vi "Main.vi"() -> ()   [LabVIEW 2014, in "ConfigurableQMH.lvlib"]
doc: "This template is based off of the Queued Message Handler design pattern and the Queued Message Handler project template that ships with LabVIEW.\n\nThe main difference is that the queue is private to this module and communication between modules is performed via Broadcast and Request events.\n\nRequest events are wrapped in public API methods and are handled in the Event Handling Loop (EHL) of this VI. Any module can register for Broadcast events sent by this module. The EHL generates messages based on user interface actions.\n\nThe Message Handling Loop (MHL) processes messages generated by the EHL, or by other messages. The messages are string values, so new messages can be added easily to the Message Cases case structure in the MHL. Each message cluster can also provide an optional value for Message Data, which is a variant that can be converted to whatever message-specific data is required.\n_____\nBased on Delacor QMH Project Template 4.0.0.47."
uses:
  ConfigurableQMH.lvlib
  <vilib>/Delacor/Delacor QMH/Libraries/Cloneable Module Admin_class/Delacor_lib_QMH_Cloneable Module Admin.lvclass
  <vilib>/LabVIEW Open Source/Configuration Manager/Manager/ConfigManager.lvclass
  <vilib>/LabVIEW Open Source Project/Unicity/UniqueName/UniqueNameClass/UniqueName.lvclass
  ModuleConfiguration--Cluster.ctl
  Module Data--cluster.ctl
  <vilib>/Delacor/Delacor QMH/Libraries/Cloneable Module Admin_class/Delacor_lib_QMH_Cloneable Module Admin.lvclass/Delacor_lib_QMH_Cloneable Module Admin.ctl
  Stop Argument--cluster.ctl
  <vilib>/Delacor/Delacor QMH/Libraries/Module Admin_class/Delacor_lib_QMH_Module Admin.lvclass/Delacor_lib_QMH_Module Admin.ctl
  GetQualifiedName Argument--cluster.ctl
  GetQualifiedName (Reply Payload)--cluster.ctl
  GetConfiguration Argument--cluster.ctl
  GetConfiguration (Reply Payload)--cluster.ctl
  Modify Configuration Argument--cluster.ctl
  <vilib>/Utility/miscctls.llb/LVPointTypeDef.ctl
  <vilib>/LabVIEW Open Source Project/Unicity/UniqueName/UniqueNameClass/UniqueName.lvclass/UniqueName.ctl
  <vilib>/Delacor/Delacor QMH/Libraries/Cloneable Module Admin_class/Delacor_lib_QMH_Get Module ID.vi
  <vilib>/Delacor/Delacor QMH/Libraries/Module Admin_class/Delacor_lib_QMH_Get External Launch.vi
  <vilib>/Delacor/Delacor QMH/Libraries/Message Queue_class/Delacor_lib_QMH_Enqueue Message (Single).vi
  <vilib>/Utility/error.llb/Error Cluster From Error Code.vi
  <vilib>/ErrorRing/Error Ring.xnode
  <vilib>/Delacor/Delacor QMH/Libraries/Message Queue_class/Delacor_lib_QMH_Message Queue.lvclass
  Clone Registration/Clone Registration.lvlib
panel:
  in  "SubModule Name":string
  in  "Launch SubModule":bool
  out "Initial Configuration":T1
  out "Current Configuration":T1
  in  "Self":refnum<class "UniqueName.lvclass">
  in  "CfgManager":refnum<class "ConfigManager.lvclass">
  in  "Simulate MHL Error":bool
  in  "Simulate EHL Error":bool
  out "error out":errorcluster
  in  "Module Admin":refnum<class "Delacor_lib_QMH_Cloneable Module Admin.lvclass">
  out "Status":string
  # "Do not modify these nodes"
  # "This template is for the a Configurable  Delacor Queued Message Handler design pattern.\n\nSee the block diagram for more information on how to use this template.\nOther QMH Modules communicate with this Module via its Public API (wrappers for its Request Events).\n\nThis Module communicates with other Modules via its Broadcast Events.\nAny module that wants to get these messages, just registers for this module's Broadcast events."
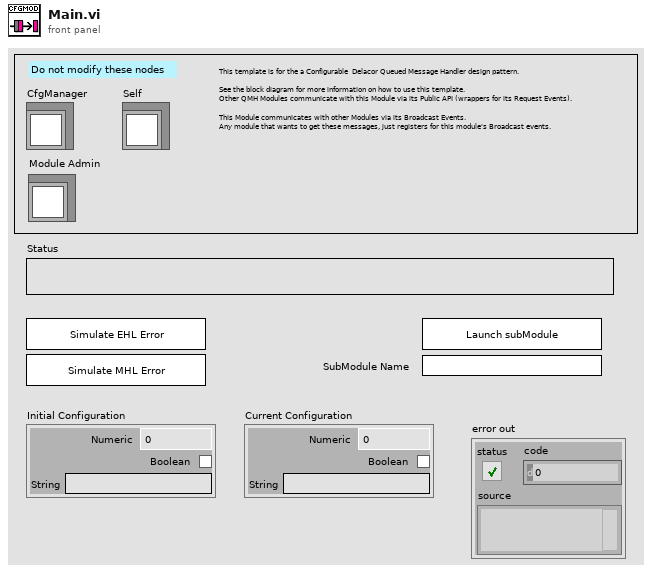
[diagram p1: front panel]
types:
  T1 = typedef "ConfigurableQMH.lvlib/ModuleConfiguration--Cluster.ctl" = cluster{"Numeric":dbl, "Boolean":bool, "String":string}
  T2 = typedef "ConfigurableQMH.lvlib/Module Data--cluster.ctl" = cluster{"Status":string, "CfgManager":refnum<class "ConfigManager.lvclass">, "Self":refnum<class "UniqueName.lvclass">, "Submodules":i32[]}
  T3 = typedef "ConfigurableQMH.lvlib/Request Events--cluster.ctl" = cluster{"Stop Module":refnum<user-event>, "Show Panel":refnum<user-event>, "Hide Panel":refnum<user-event>, "Show Diagram":refnum<user-event>, "Get Module Execution Status":refnum<user-event>, "GetQualifiedName":refnum<user-event>, "GetConfiguration":refnum<user-event>, "Modify Configuration":refnum<user-event>}
  T4 = enum32{"invalid lock state", "Not Locked", "Locked (No Password)", "Password-protected"}
  T5 = typedef "ConfigurableQMH.lvlib/Stop Argument--cluster.ctl" = cluster{"Origin":string, "Module ID":i32, "Exit via Stop Module Req?":bool, "Wait for Module to stop?":bool}
  T6 = typedef "ConfigurableQMH.lvlib/GetQualifiedName Argument--cluster.ctl" = cluster{"Module ID":i32, "Fully Qualified Name":string, "Wait Notifier":refnum<notifier>}
  T7 = typedef "ConfigurableQMH.lvlib/GetConfiguration Argument--cluster.ctl" = cluster{"Module ID":i32, "Wait Notifier":refnum<notifier>}
  T8 = typedef "ConfigurableQMH.lvlib/Modify Configuration Argument--cluster.ctl" = cluster{"Module ID":i32, "Configuration":T1}
  T9 = typedef "LVPointTypeDef.ctl" = cluster{"Horizontal":i16, "Vertical":i16}
  T10 = enum32{"Invalid", "Standard", "Closed", "Hidden", "Minimized", "Maximized"}
  T11 = typedef "ConfigurableQMH.lvlib/GetQualifiedName (Reply Payload)--cluster.ctl" = cluster{"Fully Qualified Name":string, "GetQualifiedName_error":errorcluster}
  T12 = typedef "ConfigurableQMH.lvlib/GetConfiguration (Reply Payload)--cluster.ctl" = cluster{"Configuration":T1, "GetConfiguration_error":errorcluster}
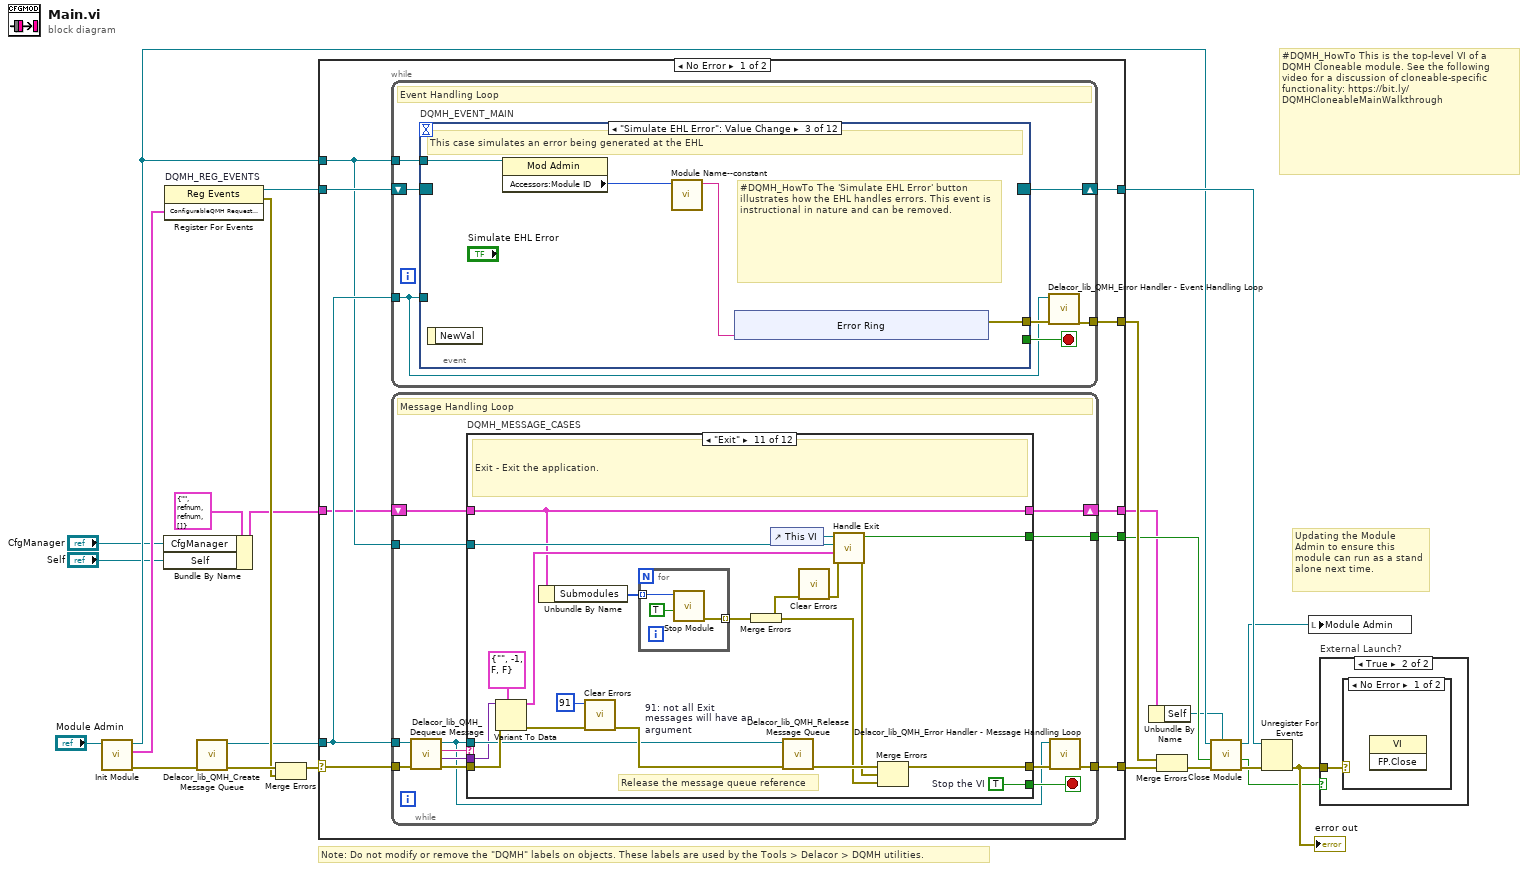
[diagram p0: block diagram]
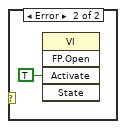
[diagram p3: hidden frame]
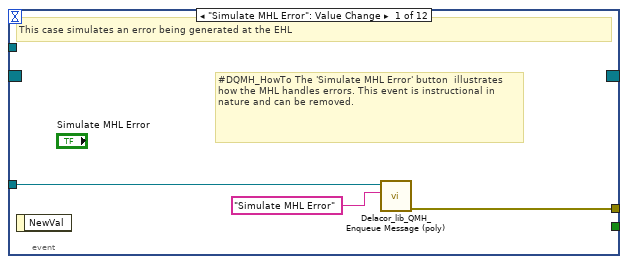
[diagram p4: hidden frame]
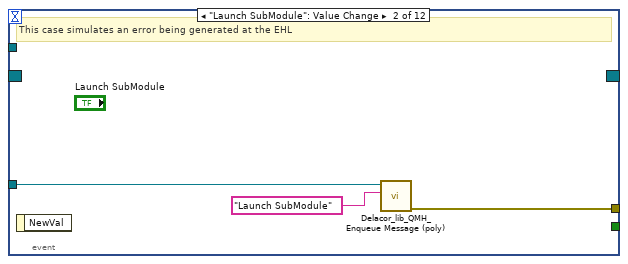
[diagram p5: hidden frame]
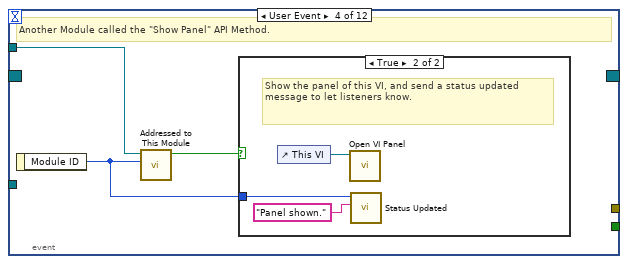
[diagram p6: hidden frame]
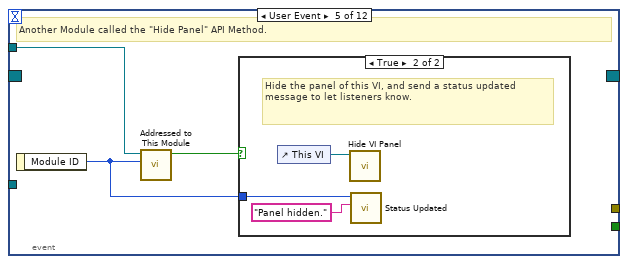
[diagram p8: hidden frame]
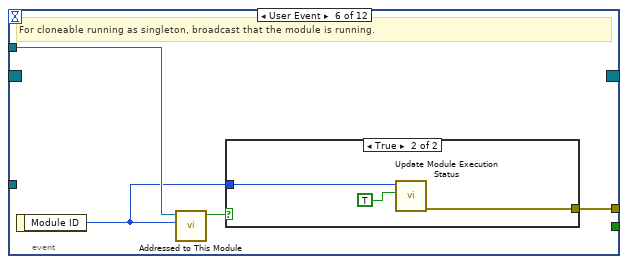
[diagram p10: hidden frame]
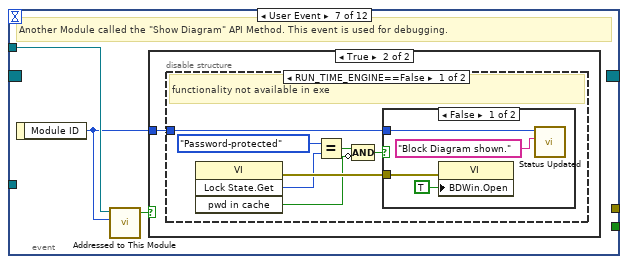
[diagram p12: hidden frame]
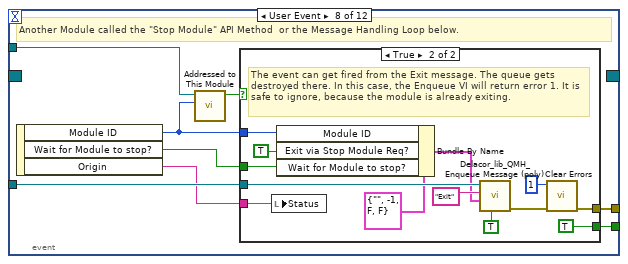
[diagram p16: hidden frame]
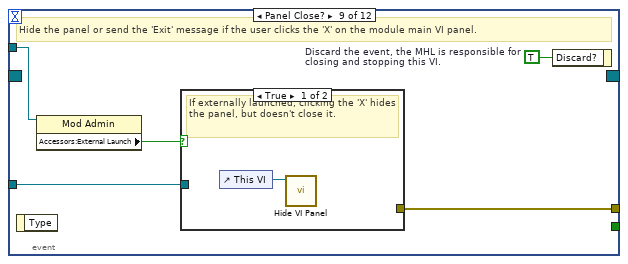
[diagram p18: hidden frame]
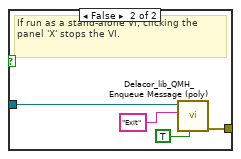
[diagram p19: hidden frame]
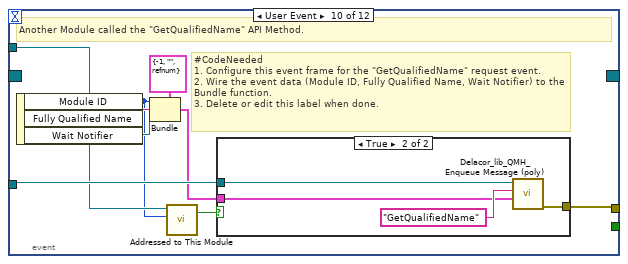
[diagram p20: hidden frame]
diagram:
  # "#DQMH_HowTo This is the top-level VI of a DQMH Cloneable module. See the following video for a discussion of cloneable-specific functionality: https://bit.ly/DQMHCloneableMainWalkthrough"
  # "Note: Do not modify or remove the \"DQMH\" labels on objects. These labels are used by the Tools > Delacor > DQMH utilities."
  # "Updating the Module Admin to ensure this module can run as a stand alone next time."
  n1 = call "Init Module.vi"("Cloneable Module Admin in"="Module Admin") -> ("error out"=w21:errorcluster, "ConfigurableQMH Request Events"=w13:T3, "Cloneable Module Admin out"=w10:refnum<class "Delacor_lib_QMH_Cloneable Module Admin.lvclass">)  [unwired: 8 in]
  n2 = Bundle By Name(cluster=T2 {"Status"="", "CfgManager"=refnum, "Self"=refnum, "Submodules"=[]} ("Data Cluster"), "CfgManager"="CfgManager", "Self"="Self") -> (w4:T2)
  n3 = register-events "DQMH_REG_EVENTS"(w13) -> (reference out=w14:refnum<event-registration>, error out=w16:errorcluster)  [unwired: 2 in]
  n4 = call <vilib>:"Delacor_lib_QMH_Create Message Queue.vi"("error in (no error)"=w21) -> ("error out"=w18:errorcluster, "Message Queue out"=w12:refnum<class "Delacor_lib_QMH_Message Queue.lvclass">)  [unwired: 9 in]
  n5 = Merge Errors(w18, w16) -> (w17:errorcluster)
  n6 = case shown="No Error" w17 {
    selector: w17 -> [w32 w339]
    tunnel: [w34 w339] -> w22
    tunnel: [w31 w338] -> w15
    tunnel: w14 -> [w30 w338]
    tunnel: w12 -> [w29 _]
    tunnel: [w33 _] -> w23
    tunnel: w10 -> [w28 w334]
    tunnel: [w27 _] -> w8
    tunnel: w4 -> [w26 w331]
    tunnel: [w25 w331] -> w1
    frame No Error {
      n7 = while {
        tunnel: w29 -> [w35]
        shift-right: [w38] -> w31
        shift-left: w30 -> [w39]
        tunnel: [w40] -> w33
        tunnel: w28 -> [w36]
        stop <- w37 stop-if-true
        # "Event Handling Loop"
        n8 = event "DQMH_EVENT_MAIN" shown="[2] \"Simulate EHL Error\": Value Change" {
          selector: w39 -> [_ _ _ _ _ _ _ _ _ _ _ _]
          dyn-events: [_ _ _ _ _ _ _ _ _ _ _ _] -> w38
          timeout: _ -> [_ _ _ _ _ _ _ _ _ _ _ _]
          tunnel: [_ _ _ _ _ _ _ w96 _ _ _ _] -> w37
          tunnel: w35 -> [w43 w46 _ _ _ _ _ w99 w115 w132 w144 w156]
          tunnel: [w44 w47 w51 _ _ w74 _ w100 w118 w127 w139 w151] -> w41
          tunnel: w36 -> [_ _ w50 w60 w66 w72 w79 w98 w116 w130 w142 w154]
          event "Simulate MHL Error": Value Change {
            # "#DQMH_HowTo The 'Simulate MHL Error' button  illustrates how the MHL handles errors. This event is instructional in nature and can be removed."
            # "This case simulates an error being generated at the EHL"
            n9 = event-data() -> ()  [unwired: 1 in, 1 out]
            n10 = call-poly <vilib>:"Delacor_lib_QMH_Enqueue Message (poly).vi"("Message"="Simulate MHL Error", "Message Queue in"=w43) -> ("error out"=w44:errorcluster)  [unwired: 8 in, 1 out]
          }
          event "Launch SubModule": Value Change {
            # "This case simulates an error being generated at the EHL"
            n11 = event-data() -> ()  [unwired: 1 in, 1 out]
            n12 = call-poly <vilib>:"Delacor_lib_QMH_Enqueue Message (poly).vi"("Message"="Launch SubModule", "Message Queue in"=w46) -> ("error out"=w47:errorcluster)  [unwired: 8 in, 1 out]
          }
          event "Simulate EHL Error": Value Change {
            # "#DQMH_HowTo The 'Simulate EHL Error' button  illustrates how the EHL handles errors. This event is instructional in nature and can be removed."
            # "This case simulates an error being generated at the EHL"
            n13 = event-data() -> ()  [unwired: 1 in, 1 out]
            n14 = property class="Mod Admin"(reference=w50) -> ("Accessors:Module ID"=w49:i32)  [unwired: 1 in, 2 out]
            n15 = call "Module Name--constant.vi"("Module ID"=w49) -> ("Module Name"=w48:string)  [unwired: 10 in]
            n16 = xnode "Error Ring"("parameter 0"=w48) -> ("error out"=w51:errorcluster)
          }
          event User Event {
            # "Another Module called the \"Show Panel\" API Method."
            n17 = event-data() -> ("Module ID"=w59:i32)  [unwired: 1 in]
            n18 = call "Addressed to This Module.vi"("Module ID from Argument"=w59, "Module Admin"=w60) -> ("Addressed to this instance?"=w61:bool)  [unwired: 8 in, 1 out]
            n19 = case shown="True" w61 {
              tunnel: w59 -> [_ w62]
              frame False {
              }
              frame True {
                # "Show the panel of this VI, and send a status updated message to let listeners know."
                n20 = control-ref of="This VI"() -> (w64:refnum<vi>)
                n21 = call "Open VI Panel.vi"("VI"=w64) -> ()  [unwired: 10 in, 1 out]
                n22 = call "Status Updated.vi"("Status"="Panel shown." ("format string"), "Module ID"=w62) -> ()  [unwired: 9 in, 1 out]
              }
            }
          }
          event User Event {
            # "Another Module called the \"Hide Panel\" API Method."
            n23 = event-data() -> ("Module ID"=w65:i32)  [unwired: 1 in]
            n24 = call "Addressed to This Module.vi"("Module ID from Argument"=w65, "Module Admin"=w66) -> ("Addressed to this instance?"=w67:bool)  [unwired: 8 in, 1 out]
            n25 = case shown="True" w67 {
              tunnel: w65 -> [_ w68]
              frame False {
              }
              frame True {
                # "Hide the panel of this VI, and send a status updated message to let listeners know."
                n26 = control-ref of="This VI"() -> (w70:refnum<vi>)
                n27 = call "Hide VI Panel.vi"("VI"=w70) -> ()  [unwired: 10 in, 1 out]
                n28 = call "Status Updated.vi"("Status"="Panel hidden." ("format string"), "Module ID"=w68) -> ()  [unwired: 9 in, 1 out]
              }
            }
          }
          event User Event {
            # "For cloneable running as singleton, broadcast that the module is running."
            n29 = event-data() -> ("Module ID"=w71:i32)  [unwired: 1 in]
            n30 = call "Addressed to This Module.vi"("Module ID from Argument"=w71, "Module Admin"=w72) -> ("Addressed to this instance?"=w73:bool)  [unwired: 8 in, 1 out]
            n31 = case shown="True" w73 {
              tunnel: [_ w77] -> w74
              tunnel: w71 -> [_ w76]
              frame False {
              }
              frame True {
                n32 = call "Update Module Execution Status.vi"("Running?"=TRUE, "Module ID"=w76) -> ("error out"=w77:errorcluster)  [unwired: 9 in]
              }
            }
          }
          event User Event {
            # "Another Module called the \"Show Diagram\" API Method. This event is used for debugging."
            n33 = event-data() -> ("Module ID"=w78:i32)  [unwired: 1 in]
            n34 = call "Addressed to This Module.vi"("Module ID from Argument"=w78, "Module Admin"=w79) -> ("Addressed to this instance?"=w80:bool)  [unwired: 8 in, 1 out]
            n35 = case shown="True" w80 {
              tunnel: w78 -> [_ w81]
              frame False {
              }
              frame True {
                n36 = disable-structure shown="RUN_TIME_ENGINE==False" {
                  disable-tunnel: w81 -> [w82 _]
                  frame condition #0 (active) {
                    # "functionality not available in exe"
                    n37 = invoke class="VI" method="Lock State.Get"() -> (error out=w88:errorcluster, "Get Lock State"=w87:T4, "pwd in cache"=w84:bool)  [unwired: 4 in, 1 out]
                    n38 = Equal?(x=T4."Password-protected", y=w87) -> (x = y?=w85:bool)
                    n39 = Compound Arithmetic op=AND(w85, invert w84) -> (w83:bool)
                    n40 = case shown="False" w83 {
                      tunnel: w88 -> [w92 _]
                      tunnel: w82 -> [w89 _]
                      frame False {
                        n41 = property class="VI"(error in=w92, "BDWin.Open"=TRUE ("Block Diagram Window:Open")) -> ()  [unwired: 1 in, 2 out]
                        n42 = call "Status Updated.vi"("Status"="Block Diagram shown." ("format string"), "Module ID"=w89) -> ()  [unwired: 9 in, 1 out]
                      }
                      frame True {
                        # "Password-protected VI, and the password is not in the cache. Do not show the diagram."
                      }
                    }
                  }
                  frame condition #1 {
                  }
                }
              }
            }
          }
          event User Event {
            # "Another Module called the \"Stop Module\" API Method  or the Message Handling Loop below."
            n43 = event-data() -> ("Module ID"=w94:i32, "Wait for Module to stop?"=w95:bool, "Origin"=w93:string)  [unwired: 1 in]
            n44 = call "Addressed to This Module.vi"("Module ID from Argument"=w94, "Module Admin"=w98) -> ("Addressed to this instance?"=w97:bool)  [unwired: 8 in, 1 out]
            n45 = case shown="True" w97 {
              tunnel: [_ w112] -> w100
              tunnel: w99 -> [_ w108]
              tunnel: [_ TRUE] -> w96
              tunnel: w95 -> [_ w103]
              tunnel: w94 -> [_ w105]
              tunnel: w93 -> [_ w101]
              frame False {
              }
              frame True {
                # "The event can get fired from the Exit message. The queue gets destroyed there. In this case, the Enqueue VI will return error 1. It is safe to ignore, because the module is already exiting."
                n46 = local write "Status"(w101) -> ()
                n47 = Bundle By Name(cluster=T5 {"Origin"="", "Module ID"=-1, "Exit via Stop Module Req?"=FALSE, "Wait for Module to stop?"=FALSE} ("Stop Argument"), "Module ID"=w105, "Exit via Stop Module Req?"=TRUE, "Wait for Module to stop?"=w103) -> (w102:T5)
                n48 = call-poly <vilib>:"Delacor_lib_QMH_Enqueue Message (poly).vi"("Priority Message? (F)"=TRUE, "Message Data"=w102, "Message"="Exit", "Message Queue in"=w108) -> ("error out"=w113:errorcluster)  [unwired: 6 in, 1 out]
                n49 = call <vilib>:"Clear Errors.vi"("error in (no error)"=w113, "specific error code to clear (0: all)"=1) -> ("error out"=w112:errorcluster)  [unwired: 4 in, 1 out]
              }
            }
          }
          event Panel Close? {
            w117 = TRUE  # Discard the event, the MHL is responsible for closing and stopping this VI.
            # "Hide the panel or send the 'Exit' message if the user clicks the 'X' on the module main VI panel."
            n50 = event-data() -> ()  [unwired: 1 in, 1 out]
            n51 = property class="Mod Admin"(reference=w116) -> ("Accessors:External Launch"=w114:bool)  [unwired: 1 in, 2 out]
            n52 = case shown="True" w114 {
              tunnel: w115 -> [_ w122]
              tunnel: [_ w123] -> w118
              frame True {
                # "If externally launched, clicking the 'X' hides the panel, but doesn't close it."
                n53 = control-ref of="This VI"() -> (w119:refnum<vi>)
                n54 = call "Hide VI Panel.vi"("VI"=w119) -> ()  [unwired: 10 in, 1 out]
              }
              frame False {
                # "If run as a stand-alone VI, clicking the panel 'X' stops the VI."
                n55 = call-poly <vilib>:"Delacor_lib_QMH_Enqueue Message (poly).vi"("Priority Message? (F)"=TRUE, "Message"="Exit", "Message Queue in"=w122) -> ("error out"=w123:errorcluster)  [unwired: 7 in, 1 out]
              }
            }
            n56 = event-data("Discard?"=w117) -> ()  [unwired: 1 in, 1 out]
          }
          event User Event {
            # "#CodeNeeded\n1. Configure this event frame for the \"GetQualifiedName\" request event.\n2. Wire the event data (Module ID, Fully Qualified Name, Wait Notifier) to the Bundle function.\n3. Delete or edit this label when done."
            # "Another Module called the \"GetQualifiedName\" API Method."
            n57 = event-data() -> ("Module ID"=w124:i32, "Fully Qualified Name"=w126:string, "Wait Notifier"=w125:refnum<notifier>)  [unwired: 1 in]
            n58 = Bundle(cluster=T6 {"Module ID"=-1, "Fully Qualified Name"="", "Wait Notifier"=refnum} ("GetQualifiedName Argument"), "Module ID"=w124, "Fully Qualified Name"=w126, "Wait Notifier"=w125) -> (w128:T6)
            n59 = call "Addressed to This Module.vi"("Module ID from Argument"=w124, "Module Admin"=w130) -> ("Addressed to this instance?"=w131:bool)  [unwired: 8 in, 1 out]
            n60 = case shown="True" w131 {
              tunnel: w132 -> [_ w136]
              tunnel: w128 -> [_ w134]
              tunnel: [_ w133] -> w127
              frame False {
              }
              frame True {
                n61 = call-poly <vilib>:"Delacor_lib_QMH_Enqueue Message (poly).vi"("Message Data"=w134, "Message"="GetQualifiedName", "Message Queue in"=w136) -> ("error out"=w133:errorcluster)  [unwired: 7 in, 1 out]
              }
            }
          }
          event User Event {
            # "Another Module called the \"GetConfiguration\" API Method."
            n62 = event-data() -> ("Module ID"=w137:i32, "Wait Notifier"=w138:refnum<notifier>)  [unwired: 1 in]
            n63 = Bundle(cluster=T7 {"Module ID"=-1, "Wait Notifier"=refnum} ("GetConfiguration Argument"), "Module ID"=w137, "Wait Notifier"=w138) -> (w140:T7)
            n64 = call "Addressed to This Module.vi"("Module ID from Argument"=w137, "Module Admin"=w142) -> ("Addressed to this instance?"=w143:bool)  [unwired: 8 in, 1 out]
            n65 = case shown="True" w143 {
              tunnel: w144 -> [_ w148]
              tunnel: w140 -> [_ w146]
              tunnel: [_ w145] -> w139
              frame False {
              }
              frame True {
                n66 = call-poly <vilib>:"Delacor_lib_QMH_Enqueue Message (poly).vi"("Message Data"=w146, "Message"="GetConfiguration", "Message Queue in"=w148) -> ("error out"=w145:errorcluster)  [unwired: 7 in, 1 out]
              }
            }
          }
          event User Event {
            # "Another Module called the \"Modify Configuration\" API Method."
            n67 = event-data() -> ("Module ID"=w149:i32, "Configuration"=w150:T1)  [unwired: 1 in]
            n68 = Bundle(cluster=T8 {"Module ID"=-1, "Configuration"={"Numeric"=0.0, "Boolean"=FALSE, "String"=""}} ("Modify Configuration Argument"), "Module ID"=w149, "Configuration"=w150) -> (w152:T8)
            n69 = call "Addressed to This Module.vi"("Module ID from Argument"=w149, "Module Admin"=w154) -> ("Addressed to this instance?"=w155:bool)  [unwired: 8 in, 1 out]
            n70 = case shown="True" w155 {
              tunnel: w156 -> [_ w160]
              tunnel: w152 -> [_ w158]
              tunnel: [_ w157] -> w151
              frame False {
              }
              frame True {
                n71 = call-poly <vilib>:"Delacor_lib_QMH_Enqueue Message (poly).vi"("Message Data"=w158, "Message"="Modify Configuration", "Message Queue in"=w160) -> ("error out"=w157:errorcluster)  [unwired: 7 in, 1 out]
              }
            }
          }
        }
        n72 = call-dynamic "Delacor_lib_QMH_Error Handler - Event Handling Loop.vi"("error in (no error)"=w41, "Message Queue in"=w35) -> ("dup error in"=w40:errorcluster)  [unwired: 8 in, 1 out]
      }
      n73 = while {
        tunnel: w29 -> [w164]
        shift-right: [w168] -> w25
        shift-left: w26 -> [w169]
        tunnel: w32 -> [w172]
        tunnel: [w170] -> w34
        tunnel: w28 -> [w162]
        tunnel: [w161] -> w27
        stop <- w167 stop-if-true
        # "Message Handling Loop"
        n74 = call-dynamic "Delacor_lib_QMH_Dequeue Message.vi"("error in (no error)"=w172, "Message Queue in"=w164) -> ("error out"=w171:errorcluster, "Message Data"=w165:variant, "Message"=w166:string, "Message Queue out"=w163:refnum<class "Delacor_lib_QMH_Message Queue.lvclass">)  [unwired: 6 in]
        n75 = case "DQMH_MESSAGE_CASES" shown="\"Exit\"" w166 {
          selector: w166 -> [_ _ _ _ _ _ _ _ _ _ _ w318]
          tunnel: w163 -> [_ _ _ _ _ _ _ _ w261 _ w305 _]
          tunnel: w171 -> [w200 w204 w220 w232 w243 w252 w258 w260 w271 w284 w311 w320]
          tunnel: [w182 w204 w209 w224 w237 w250 w257 w260 w267 w283 w308 w321] -> w173
          tunnel: w169 -> [w176 w203 w214 w223 w239 w248 w256 w259 w266 w281 w296 w319]
          tunnel: [w192 w203 w214 w222 w238 w247 w256 w259 w266 w281 w296 w319] -> w168
          tunnel: [_ _ _ _ _ _ _ _ _ _ w304 _] -> w167
          tunnel: w165 -> [_ _ w219 w231 w242 _ _ _ w265 _ w302 _]
          tunnel: w162 -> [w188 _ _ _ _ _ _ _ w264 w279 w298 w316]
          tunnel: [_ _ _ _ _ _ _ _ _ _ w300 _] -> w161
          frame "Initialize" {
            w186 = "Initial Message" ("Initial Message")
            # "THIS OVERRIDES THE\nCONFIG FOR DEMO PURPOSES.\nREMOVE IT."
            # "Initialize - Any operation that needs to be done before the module can receive messages. Synchronize Caller Events.vi will inform Start Module.vi that the module has launched and is ready to receive messages. Module Did Init.vi will broadcast that the module initialized."
            n76 = call "Synchronize Caller Events.vi"("error in (no error)"=w200, "Module Admin"=w188) -> ("error out"=w199:errorcluster, "Module Admin out"=w177:refnum<class "Delacor_lib_QMH_Cloneable Module Admin.lvclass">)  [unwired: 8 in]
            n77 = Unbundle By Name(w176) -> ("Self"=w175:refnum<class "UniqueName.lvclass">)
            n78 = call <vilib>:"Read UUID.vi"("UniqueName in"=w175) -> ("UUID"=w174:string)  [unwired: 9 in, 1 out]
            n79 = property class="Mod Admin"(reference=w177) -> ("Accessors:Module ID"=w181:i32, "Accessors:External Launch"=w189:bool)  [unwired: 1 in, 2 out]
            n80 = Random Number (0-1)() -> (number: 0 to 1=w185:dbl)
            n81 = call "Get Module Configuration.vi"("Data Cluster"=w176) -> ("Configuration"=w184:T1, "Data Cluster dup"=w180:T2)  [unwired: 8 in, 1 out]
            n82 = Bundle By Name(cluster=w184, "Numeric"=w185, "String"=w174) -> (w178:T1)
            "Initial Configuration" <- w178
            n83 = call "Module Name--constant.vi"("Module ID"=w181) -> ("Module Name"=w196:string)  [unwired: 10 in]
            n84 = local write "Current Configuration"(w178) -> ()
            n85 = call "Set Module Configuration.vi"("Configuration"=w178, "Data Cluster"=w180) -> ("Data Cluster dup"=w179:T2)  [unwired: 8 in, 1 out]
            n86 = call "Module Name--constant.vi"("Module ID"=w181) -> ("Module Name"=w190:string)  [unwired: 10 in]
            n87 = property class="VI"("Front Panel.Title"=w196) -> (reference out=w198:refnum<vi>, error out=w202:errorcluster)  [unwired: 2 in]
            n88 = Select(t=T10."Hidden" ("State"), s=w189, f=T10."Standard" ("State")) -> (s? t:f=w193:T10)
            n89 = call "Module Did Init.vi"("error in (no error)"=w199, "Initialized?"=TRUE, "Origin"=w190, "Module ID"=w181) -> ("error out"=w183:errorcluster)  [unwired: 7 in]
            n90 = invoke class="VI" method="FP.Open"(reference=w198, error in=w202, "State"=w193) -> (reference out=w197:refnum<vi>, error out=w201:errorcluster)  [unwired: 2 in, 3 out]
            n91 = Bundle By Name(cluster=w179, "Status"=w186) -> (w192:T2)
            n92 = invoke class="VI" method="FP.Center"(reference=w197, error in=w201) -> ()  [unwired: 1 in, 3 out]
            n93 = property on="Pane" class="Pane"("Origin"=T9 {"Horizontal"=0, "Vertical"=0}) -> ()  [unwired: 2 in, 2 out]
            n94 = call "Module Configuration.vi"("error in (no error)"=w183, "Configuration"=w178, "Module ID"=w181) -> ("error out"=w182:errorcluster)  [unwired: 8 in]
            "Status" <- w186
          }
          frame "--- Module Specific ---" {
            # "Separator -- The following cases handle messages specific to this Module."
          }
          frame "GetQualifiedName" {
            # "Requests the module's Fully Qualified Name"
            n95 = Unbundle By Name(w214) -> ("Self"=w213:refnum<class "UniqueName.lvclass">)
            n96 = Variant To Data(error in=w220, type=T6 {"Module ID"=-1, "Fully Qualified Name"="", "Wait Notifier"=refnum} ("GetQualifiedName Argument"), Variant=w219) -> (data=w217:T6, error out=w208:errorcluster)
            n97 = call <vilib>:"Read Fully Qualified Name.vi"("UniqueName in"=w213) -> ("Fully Qualified Name"=w207:string)  [unwired: 9 in, 1 out]
            n98 = Unbundle By Name(w217) -> ("Wait Notifier"=w215:refnum<notifier>, "Module ID"=w211:i32)
            n99 = Bundle By Name(cluster=T11 {"Fully Qualified Name"="", "GetQualifiedName_error"={"status"=FALSE, "code"=0, "source"=""}} ("GetQualifiedName (Reply Payload)"), "Fully Qualified Name"=w207) -> (w216:T11)
            n100 = Format Into String(format string="FQN: %s", w207) -> (resulting string=w206:string)  [unwired: 2 in, 1 out]
            n101 = Send Notification(notification=w216, notifier=w215, error in (no error)=w208) -> (error out=w210:errorcluster)  [unwired: 1 out]
            n102 = call "Status Updated.vi"("error in (no error)"=w210, "Status"=w206, "Module ID"=w211) -> ("error out"=w209:errorcluster)  [unwired: 8 in]
          }
          frame "GetConfiguration" {
            n103 = Variant To Data(error in=w232, type=T7 {"Module ID"=-1, "Wait Notifier"=refnum} ("GetConfiguration Argument"), Variant=w231) -> (data=w229:T7, error out=w225:errorcluster)
            n104 = call "Get Module Configuration.vi"("error in (no error)"=w225, "Data Cluster"=w223) -> ("error out"=w224:errorcluster, "Configuration"=w221:T1, "Data Cluster dup"=w222:T2)  [unwired: 7 in]
            "Current Configuration" <- w221
            n105 = Unbundle By Name(w229) -> ("Wait Notifier"=w228:refnum<notifier>)
            n106 = Bundle By Name(cluster=T12 {"Configuration"={"Numeric"=0.0, "Boolean"=FALSE, "String"=""}, "GetConfiguration_error"={"status"=FALSE, "code"=0, "source"=""}} ("GetConfiguration (Reply Payload)"), "Configuration"=w221, "GetConfiguration_error"=w224) -> (w227:T12)
            n107 = Send Notification(notification=w227, notifier=w228) -> ()  [unwired: 1 in, 2 out]
          }
          frame "Modify Configuration" {
            n108 = Variant To Data(error in=w243, type=T8 {"Module ID"=-1, "Configuration"={"Numeric"=0.0, "Boolean"=FALSE, "String"=""}} ("Modify Configuration Argument"), Variant=w242) -> (data=w240:T8, error out=w234:errorcluster)
            n109 = Unbundle By Name(w240) -> ("Configuration"=w235:T1, "Module ID"=w236:i32)
            n110 = call "Set Module Configuration.vi"("error in (no error)"=w234, "Configuration"=w235, "Data Cluster"=w239) -> ("error out"=w233:errorcluster, "Data Cluster dup"=w238:T2)  [unwired: 7 in]
            n111 = local write "Current Configuration"(w235) -> ()
            n112 = call "Module Configuration.vi"("error in (no error)"=w233, "Configuration"=w235, "Module ID"=w236) -> ("error out"=w237:errorcluster)  [unwired: 8 in]
          }
          frame "Launch SubModule" {
            n113 = Unbundle By Name(w248) -> ("Submodules"=w246:i32[], "CfgManager"=w255:refnum<class "ConfigManager.lvclass">, "Self"=w254:refnum<class "UniqueName.lvclass">)
            n114 = call "Start Module.vi"("CfgManager"=w255, "error in (no error)"=w252, "Owner"=w254, "Module Name (empty: default)"="SubModule Name") -> ("error out"=w251:errorcluster, "Wait for Event Sync?"=w249:bool, "Module ID"=w245:i32)  [unwired: 4 in, 1 out]
            n115 = Build Array (concatenate)(w246, w245) -> (w244:i32[])
            n116 = Bundle By Name(cluster=w248, "Submodules"=w244) -> (w247:T2)
            n117 = call "Synchronize Module Events.vi"("error in (no error)"=w251, "Wait for Event Sync?"=w249, "Module ID"=w245) -> ("error out"=w250:errorcluster)  [unwired: 7 in, 1 out]
          }
          frame "---Copy This Frame---" {
            # "Duplicate this frame when creating new messages.  Change this comment in the duplicated frame to describe this message."
            n118 = Merge Errors(w258) -> (w257:errorcluster)
          }
          frame "--- Exit and Error Handling---" {
            # "Separator - the following cases handle errors and exit messages."
          }
          frame "Error" {
            # "#CodeRecommended - If you ever change the name of this \"Error\" message, you'll need to update the name in the Check Loop Error.vi as well."
            # "#CodeRecommended - If the module is running in standalone mode (External Launch = FALSE), this code will pop up an error dialog and call the 'Exit' message if an error occurs. Add more fine-grained error handling here."
            # "Error - Check the error message data and respond accordingly. This message is sent by the \"Error Handler\" VIs at the end of each loop in this application."
            n119 = property class="Mod Admin"(reference=w264) -> ("Accessors:External Launch"=w262:bool, "Accessors:Module ID"=w263:i32)  [unwired: 1 in, 2 out]
            n120 = Variant To Data(error in=w271, type=errorcluster {"status"=FALSE, "code"=0, "source"=""} ("error constant"), Variant=w265) -> (data=w272:errorcluster, error out=w269:errorcluster)
            n121 = call "Error Reported.vi"("Error"=w272, "Module ID"=w263) -> ()  [unwired: 9 in, 1 out]
            n122 = case shown="False" w262 {
              tunnel: [w277 _] -> w268
              tunnel: w261 -> [w275 _]
              tunnel: w272 -> [w276 _]
              frame False {
                # "If the module is running standalone, then pop up an error dialog and call the \"Exit\" message."
                n123 = call <vilib>:"Simple Error Handler.vi"("error in (no error)"=w276) -> ()  [unwired: 4 in, 5 out]
                n124 = call-poly <vilib>:"Delacor_lib_QMH_Enqueue Message (poly).vi"("Priority Message? (F)"=TRUE, "Message"="Exit", "Message Queue in"=w275) -> ("error out"=w277:errorcluster)  [unwired: 7 in, 1 out]
              }
              frame True {
                # "If the module was launched externally, calling the Error Reported broadcast VI is the only action performed by the \"Error\" message. The module's caller can then process the error appropriately."
              }
            }
            n125 = Merge Errors(w269, w268) -> (w267:errorcluster)
            n126 = local write "error out"(w267) -> ()
          }
          frame "Simulate MHL Error" {
            # "#DQMH_HowTo The 'Simulate MHL Error' button  illustrates how the MHL handles errors. This event is instructional in nature and can be removed."
            # "Simulate an error occurring at the MHL"
            n127 = property class="Mod Admin"(reference=w279) -> ("Accessors:Module ID"=w280:i32)  [unwired: 1 in, 2 out]
            n128 = call "Module Name--constant.vi"("Module ID"=w280) -> ("Module Name"=w278:string)  [unwired: 10 in]
            n129 = xnode "Error Ring"("parameter 0"=w278) -> ("error out"=w282:errorcluster)
            n130 = Merge Errors(w284, w282) -> (w283:errorcluster)
          }
          frame "Exit" {
            w303 = 91  # 91: not all Exit messages will have an argument
            w304 = TRUE  # Stop the VI
            # "Release the message queue reference"
            # "Exit - Exit the application."
            n131 = Variant To Data(error in=w311, type=T5 {"Origin"="", "Module ID"=-1, "Exit via Stop Module Req?"=FALSE, "Wait for Module to stop?"=FALSE} ("Stop Argument"), Variant=w302) -> (data=w299:T5, error out=w306:errorcluster)
            n132 = Unbundle By Name(w296) -> ("Submodules"=w295:i32[])
            n133 = call <vilib>:"Clear Errors.vi"("error in (no error)"=w306, "specific error code to clear (0: all)"=w303) -> ("error out"=w310:errorcluster)  [unwired: 4 in, 1 out]
            n134 = for {
              tunnel: w295 -> [w314] mode=indexing
              tunnel: [w312] -> w294 mode=indexing
              n135 = call "Stop Module.vi"("Wait for Module to stop? (F)"=TRUE, "Module ID"=w314) -> ("error out"=w312:errorcluster)  [unwired: 9 in]
            }
            n136 = Merge Errors(w294) -> (w292:errorcluster)
            n137 = control-ref of="This VI"() -> (w297:refnum<vi>)
            n138 = call-dynamic "Delacor_lib_QMH_Release Message Queue.vi"("error in (no error)"=w310, "Message Queue"=w305) -> ("error out"=w309:errorcluster)  [unwired: 9 in]
            n139 = call <vilib>:"Clear Errors.vi"("error in (no error)"=w292) -> ("error out"=w293:errorcluster)  [unwired: 5 in, 1 out]
            n140 = call "Handle Exit.vi"("error in (no error)"=w293, "Stop Argument"=w299, "Module Admin in"=w298, "VI reference"=w297) -> ("error out"=w307:errorcluster, "Wait for Stop?"=w300:bool)  [unwired: 6 in]
            n141 = Merge Errors(w309, w307, w292) -> (w308:errorcluster)
          }
          frame Default {
            # "'Default' case only runs if there is a message that isn't defined in any of the other cases.  Output a programming error."
            n142 = property class="Mod Admin"(reference=w316) -> ("Accessors:Module ID"=w315:i32)  [unwired: 1 in, 2 out]
            n143 = call "Module Name--constant.vi"("Module ID"=w315) -> ("Module Name"=w317:string)  [unwired: 10 in]
            n144 = xnode "Error Ring"("parameter 0"=w318, "parameter 1"=w317) -> ("error out"=w322:errorcluster)
            n145 = Merge Errors(w320, w322) -> (w321:errorcluster)
          }
        }
        n146 = call-dynamic "Delacor_lib_QMH_Error Handler - Message Handling Loop.vi"("error in (no error)"=w173, "Message Queue in"=w163) -> ("dup error in"=w170:errorcluster)  [unwired: 8 in, 1 out]
      }
    }
    frame Error {
      n147 = call "Synchronize Caller Events.vi"("Module Admin"=w334) -> ("Module Admin out"=w333:refnum<class "Delacor_lib_QMH_Cloneable Module Admin.lvclass">)  [unwired: 9 in, 1 out]
      n148 = property class="Mod Admin"(reference=w333) -> ("Accessors:Module ID"=w332:i32)  [unwired: 1 in, 2 out]
      n149 = call "Module Name--constant.vi"("Module ID"=w332) -> ("Module Name"=w337:string)  [unwired: 10 in]
      n150 = call "Remove.vi"("Module ID"=w332) -> ()  [unwired: 9 in, 2 out]
      n151 = Format Into String(format string="An error occurred during initialization. %s is no longer running.", w337) -> (resulting string=w335:string)  [unwired: 2 in, 1 out]
      n152 = call "Error Reported.vi"("Additional Information"=w335, "Error"=w339, "Module ID"=w332) -> ()  [unwired: 8 in, 1 out]
    }
  }
  n153 = Unbundle By Name(w1) -> ("Self"=w2:refnum<class "UniqueName.lvclass">)
  n154 = Merge Errors(w23, w22) -> (w24:errorcluster)
  n155 = call "Close Module.vi"("Self"=w2, "error in (no error)"=w24, "Wait for stop?"=w8, "Module Admin in"=w10) -> ("error out"=w20:errorcluster, "External Launch"=w7:bool, "Module Admin out"=w9:refnum<class "Delacor_lib_QMH_Cloneable Module Admin.lvclass">)  [unwired: 5 in]
  n156 = Unregister For Events(event registration refnum=w15, error in=w20) -> (error out=w19:errorcluster)
  "error out" <- w19
  n157 = local write "Module Admin"(w9) -> ()
  n158 = case "External Launch?" shown="True" w7 {
    tunnel: w19 -> [_ w340]
    frame False {
    }
    frame True {
      n159 = case shown="No Error" w340 {
        frame No Error {
          n160 = invoke class="VI" method="FP.Close"() -> ()  [unwired: 3 in, 3 out]
        }
        frame Error {
          n161 = invoke class="VI" method="FP.Open"("Activate"=TRUE ("Activate?")) -> ()  [unwired: 4 in, 5 out]
        }
      }
    }
  }
